vi "KE2410_Test.vi"(8 "error in (no error)":errorcluster, 11 "KE2410 in":refnum<class "KE2410.lvclass">) -> (0 "error out":errorcluster, 3 "KE2410 out":refnum<class "KE2410.lvclass">)   [LabVIEW 2018, in "KE2410.lvclass"]
uses:
  KE2410.lvclass
  <vilib>/Platform/TimedLoop/XDataNode/timing_clust.ctl
  <vilib>/Platform/TimedLoop/XDataNode/nitl_modes.ctl
  <vilib>/Platform/TimedLoop/XDataNode/wakeup.ctl
  InstrumentSetup.vi
  <vilib>/platform/TimedLoop/XDataNode/XDataNode.xnode
  <vilib>/Platform/TimedLoop/XDataNode/XDNodeRunTimeDep.lvlib
  InstrControl.lvclass
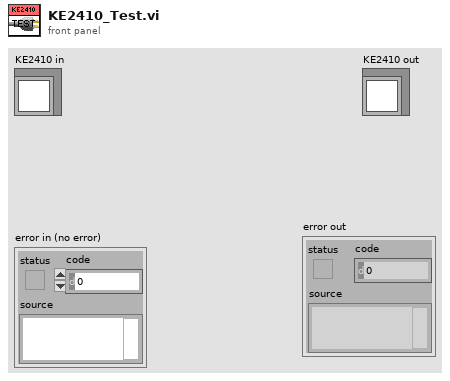
[diagram p1: front panel]
types:
  T1 = cluster{"KE 2410":cluster{"Instrument name":string, "GPIB address":string, "Instrument type":u16}, "KE 6517":cluster{"Instrument name":string, "GPIB address":string, "Instrument type":u16}, "KE 487":cluster{"Instrument name":string, "GPIB address":string, "Instrument type":u16}, "KE 2657A":cluster{"Instrument name":string, "GPIB address":string, "Instrument type":u16}, "KE 236":cluster{"Instrument name":string, "GPIB address":string, "Instrument type":u16}, "WK 6440B":cluster{"Instrument name":string, "GPIB address":string, "Instrument type":u16}, "WK 6425":cluster{"Instrument name":string, "GPIB address":string, "Instrument type":u16}, "Pickering Matrix":cluster{"Instrument name":string, "GPIB address":string, "Instrument type":u16}, "KE 2000":cluster{"Instrument name":string, "GPIB address":string, "Instrument type":u16}}
  T2 = typedef "XDNodeRunTimeDep.lvlib/timing_clust.ctl" = cluster{"Expected End [f-1]":u64, "Actual End [f-1]":u64, "Finished Late? [f-1]":bool, "Expected End [i-1]":u64, "Actual End [i-1]":u64, "Finished Late? [i-1]":bool, "Expected Start [i]":u64, "Actual Start [i]":u64, "Expected Start [f]":u64, "Actual Start [f]":u64, "Source Name":string, "Structure Name":string, "Period":i64, "Deadline":i64, "Offset":i64, "Start":i64, "Priority":i32, "Timeout":i32, "Mode":T3, "Wakeup Reason":T4, "Error":errorcluster, "Source Type":string, "Secondary Source Type":string, "Global End Time":u64, "Global Start Time":u64, "Frame Duration":u64, "Iteration Duration":u64, "Assigned CPU":i32, "I/O Scan Engine Mode":u32}
  T3 = typedef "XDNodeRunTimeDep.lvlib/nitl_modes.ctl" = enum32{"No Change", "Process missed periods, maintain original phase", "Discard missed periods, maintain original phase", "Process missed periods, ignore original phase", "Discard missed periods, ignore original phase"}
  T4 = typedef "XDNodeRunTimeDep.lvlib/wakeup.ctl" = enum32{"Normal", "Aborted", "Asynchronous wakeup", "Timing source error", "Timed loop error", "Timeout"}
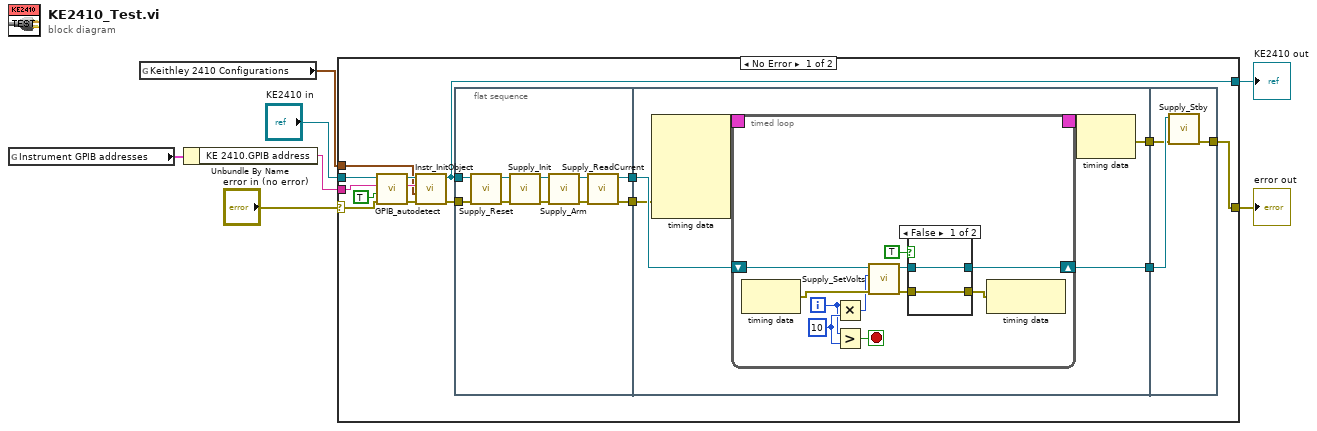
[diagram p0: block diagram]
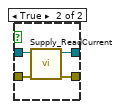
[diagram p2: hidden frame]
diagram:
  n1 = global read "InstrumentSetup.vi" "Instrument GPIB addresses"() -> (w3:T1)
  n2 = global read "InstrumentSetup.vi" "Keithley 2410 Configurations"() -> (w1:cluster{"Current Limit":sgl})
  n3 = Unbundle By Name(w3) -> ("KE 2410.GPIB address"=w2:string)
  n4 = case shown="No Error" "error in (no error)" {
    selector: "error in (no error)" -> [w15 w70]
    tunnel: "KE2410 in" -> [w12 w69]
    tunnel: [w18 w69] -> w6
    tunnel: [w17 w70] -> w5
    tunnel: w2 -> [w13 _]
    tunnel: w1 -> [w9 _]
    frame No Error {
      n5 = call-dynamic "GPIB_autodetect.vi"("error in (no error)"=w15, "Verify GPIB address"=TRUE, "Instrument GPIB address in"=w13, "InstrControl in"=w12) -> ("error out"=w14:errorcluster, "Instrument GPIB address"=w10:string, "InstrControl out"=w11:refnum<class "KE2410.lvclass">)  [unwired: 5 in]
      n6 = call-dynamic "Instr_InitObject.vi"("error in (no error)"=w14, "Instrument Configuration"=w9, "GPIB address"=w10, "KE2410 in"=w11) -> ("error out"=w19:errorcluster, "KE2410 out"=w18:refnum<class "KE2410.lvclass">)  [unwired: 6 in]
      n7 = flat-sequence {
        tunnel: w19 -> [w27]
        tunnel: w18 -> [w26]
        tunnel: [w24] -> w22
        tunnel: [w23] -> w16
        tunnel: w22 -> [w38]
        tunnel: [w37] -> w21
        tunnel: [w34] -> w20
        tunnel: w16 -> [w33]
        tunnel: [w66] -> w17
        tunnel: w21 -> [w67]
        tunnel: w20 -> [w68]
        frame #0 {
          n8 = call-dynamic "Supply_Reset.vi"("error in (no error)"=w27, "SupplyControl in"=w26) -> ("error out"=w31:errorcluster, "SupplyControl out"=w25:refnum<class "KE2410.lvclass">)  [unwired: 8 in]
          n9 = call-dynamic "Supply_Init.vi"("error in (no error)"=w31, "SupplyControl in"=w25) -> ("error out"=w30:errorcluster, "SupplyControl out"=w32:refnum<class "KE2410.lvclass">)  [unwired: 8 in]
          n10 = call-dynamic "Supply_Arm.vi"("error in (no error)"=w30, "SupplyControl in"=w32) -> ("error out"=w28:errorcluster, "SupplyControl out"=w29:refnum<class "KE2410.lvclass">)  [unwired: 8 in]
          n11 = call-dynamic "Supply_ReadCurrent.vi"("error in (no error)"=w28, "SupplyControl in"=w29) -> ("error out"=w23:errorcluster, "SupplyControl out"=w24:refnum<class "KE2410.lvclass">)  [unwired: 7 in, 1 out]
        }
        frame #1 {
          n12 = node-c288(w33) -> (w36:T2)  [unwired: 4 in]
          n13 = timed-loop {
            timing: w36 -> [_]
            timing-out: [_] -> w35
            shift-right: [w41] -> w34
            shift-left: w38 -> [w47]
            i -> [w45]
            stop <- w44 stop-if-true
            w46 = 10
            n14 = node-c288() -> (w49:errorcluster)  [unwired: 1 in]
            n15 = Multiply(x=w45, y=w46) -> (x*y=w48:i32)
            n16 = Greater?(x=w45, y=w46) -> (0:w44:bool)
            n17 = call-dynamic "Supply_SetVolts.vi"("error in (no error)"=w49, "Volts IN [V]"=w48, "KE2410 in"=w47) -> ("error out"=w43:errorcluster, "KE2410 out"=w42:refnum<class "KE2410.lvclass">)  [unwired: 6 in, 1 out]
            n18 = case shown="False" TRUE {
              tunnel: w43 -> [w51 w55]
              tunnel: w42 -> [w50 w54]
              tunnel: [w50 w53] -> w41
              tunnel: [w51 w52] -> w40
              frame False {
              }
              frame True {
                n19 = call-dynamic "Supply_ReadCurrent.vi"("error in (no error)"=w55, "SupplyControl in"=w54) -> ("error out"=w52:errorcluster, "SupplyControl out"=w53:refnum<class "KE2410.lvclass">)  [unwired: 7 in, 1 out]
              }
            }
            n20 = node-c288(w40) -> ()  [unwired: 1 out]
          }
          n21 = node-c288(w35) -> (w37:errorcluster)
        }
        frame #2 {
          n22 = call-dynamic "Supply_Stby.vi"("error in (no error)"=w67, "SupplyControl in"=w68) -> ("error out"=w66:errorcluster)  [unwired: 8 in, 1 out]
        }
      }
    }
    frame Error {
    }
  }
  "error out" <- w5
  "KE2410 out" <- w6
